vi "Setup.vi"(9 "Active Project":refnum<vi>, 10 "NI.LV.Dialog Instance":refnum<vi>) -> (2 "Target":string, 3 "_Rescript Msg out":refnum<class "_Msg Rescript.lvclass">)   [LabVIEW 2025, in "_Msg Rescript.lvlib" / "_Msg Rescript.lvclass"]
uses:
  _Msg Rescript.lvclass
  _Msg Rescript.lvclass/_Msg Rescript.ctl
  _Shared/Project Stuff/Project Stuff.lvclass
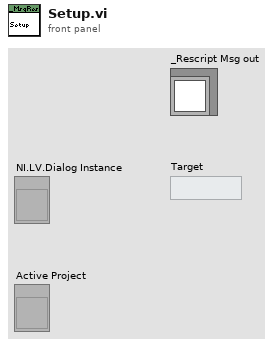
[diagram p1: front panel]
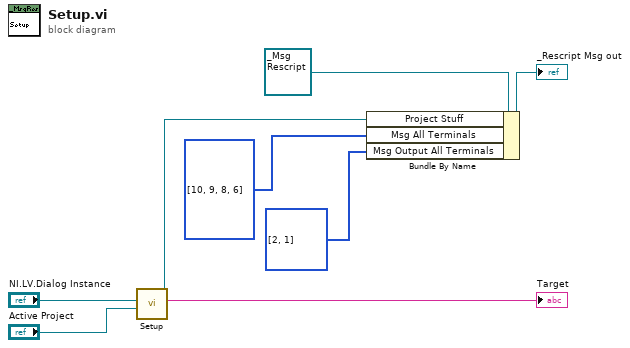
[diagram p0: block diagram]
diagram:
  n1 = call "Setup.vi"("Active Project"="Active Project", "NI.LV.Dialog Instance"="NI.LV.Dialog Instance") -> ("Target"=→"Target":string, "Project Stuff out"=w4:refnum<class "Project Stuff.lvclass">)  [unwired: 8 in]
  n2 = Bundle By Name(cluster=refnum<class "_Msg Rescript.lvclass"> refnum ("_Rescript Msg out"), "Project Stuff"=w4, "Msg All Terminals"=i32[] [10, 9, 8, 6] ("Msg Control"), "Msg Output All Terminals"=i32[] [2, 1] ("Msg Output Indicator")) -> (→"_Rescript Msg out":refnum<class "_Msg Rescript.lvclass">)
